vi "startSweepAndWait.vi"(8 "error in (no error)":errorcluster, 10 "time (s) [10 s]":dbl=10.0, 11 "Instrument.LockinAPI in":refnum<class "Instrument.LockinAPI.lvclass">) -> (0 "error out":errorcluster, 3 "Instrument.LockinAPI out":refnum<class "Instrument.LockinAPI.lvclass">)   [LabVIEW 2019, in "Instrument.LockinAPI.lvclass"]
uses:
  Instrument.LockinAPI.lvclass
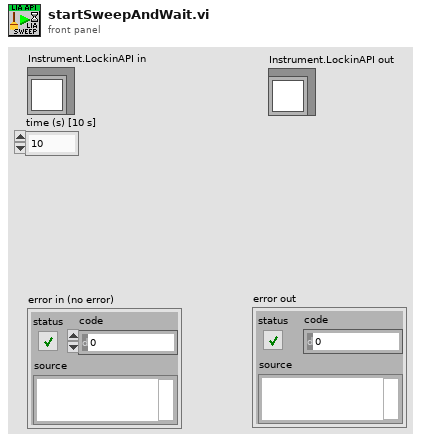
[diagram p1: front panel]
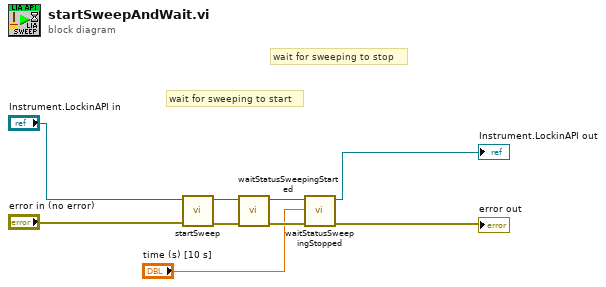
[diagram p0: block diagram]
diagram:
  # "wait for sweeping to stop"
  # "wait for sweeping to start"
  n1 = call-dynamic "startSweep.vi"("error in (no error)"="error in (no error)", "Instrument.LockinAPI in"="Instrument.LockinAPI in") -> ("error out"=w4:errorcluster, "Instrument.LockinAPI out"=w7:refnum<class "Instrument.LockinAPI.lvclass">)  [unwired: 8 in]
  n2 = call-dynamic "waitStatusSweepingStarted.vi"("error in (no error)"=w4, "Instrument.LockinAPI in"=w7) -> ("error out"=w5:errorcluster, "Instrument.LockinAPI out"=w6:refnum<class "Instrument.LockinAPI.lvclass">)  [unwired: 8 in]
  n3 = call-dynamic "waitStatusSweepingStopped.vi"("error in (no error)"=w5, "time (s) [10 s]"="time (s) [10 s]", "Instrument.LockinAPI in"=w6) -> ("error out"=→"error out":errorcluster, "Instrument.LockinAPI out"=→"Instrument.LockinAPI out":refnum<class "Instrument.LockinAPI.lvclass">)  [unwired: 7 in]
